vi "Set Power.vi"(8 "error in (no error)":errorcluster, 10 "Power":dbl, 11 "Lauda Settings":T1) -> (0 "error out":errorcluster, 1 "Connection Error":bool, 3 "Lauda Settings":T1)   [LabVIEW 2018, in "Lauda TCU.lvlib"]
uses:
  Lauda TCU.lvlib
  Lauda Settings.ctl
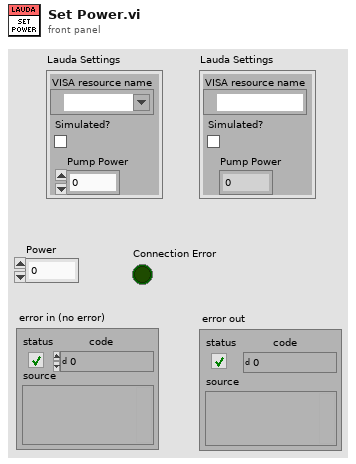
[diagram p1: front panel]
types:
  T1 = typedef "Lauda TCU.lvlib/Lauda Settings.ctl" = cluster{"VISA resource name":refnum<visa-resource-name>, "Simulated?":bool, "Pump Power":i32}
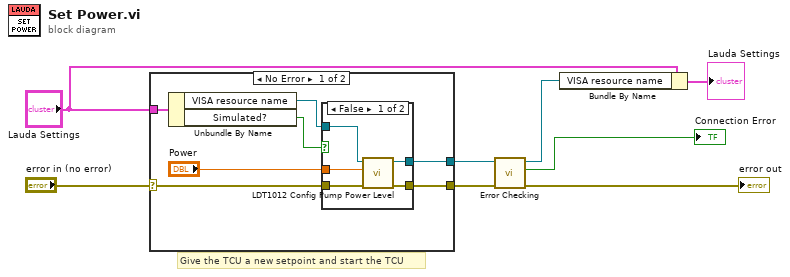
[diagram p0: block diagram]
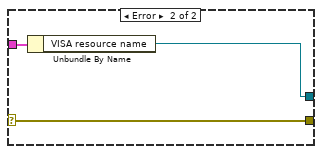
[diagram p3: hidden frame]
diagram:
  # "Give the TCU a new setpoint and start the TCU"
  n1 = case shown="No Error" "error in (no error)" {
    selector: "error in (no error)" -> [w15 w25]
    tunnel: "Lauda Settings" -> [w11 w24]
    tunnel: [w14 w25] -> w6
    tunnel: [w13 w23] -> w7
    frame No Error {
      n2 = Unbundle By Name(w11) -> ("VISA resource name"=w9:refnum<visa-resource-name>, "Simulated?"=w12:bool)
      n3 = case shown="False" w12 {
        tunnel: w15 -> [w18 w22]
        tunnel: [w17 w22] -> w14
        tunnel: [w16 w21] -> w13
        tunnel: w9 -> [w19 w21]
        tunnel: "Power" -> [w20 _]
        frame False {
          n4 = call "LDT1012 Config Pump Power Level.vi"("error in (no error)"=w18, "Pump Power Level (2: Default)"=w20, "VISA session"=w19) -> ("error out"=w17:errorcluster, "dup VISA session"=w16:refnum<visa-resource-name>)  [unwired: 7 in]
        }
        frame True {
        }
      }
    }
    frame Error {
      n5 = Unbundle By Name(w24) -> ("VISA resource name"=w23:refnum<visa-resource-name>)
    }
  }
  n6 = call "Error Checking.vi"("error in (no error)"=w6, "VISA resource name"=w7) -> ("error out"=→"error out":errorcluster, "Connection Error"=→"Connection Error":bool, "VISA resource name"=w4:refnum<visa-resource-name>)  [unwired: 7 in]
  n7 = Bundle By Name(cluster="Lauda Settings", "VISA resource name"=w4) -> (→"Lauda Settings":T1)
